vi "Array2DLastNColumns.vi"(2 "Array in":dbl[][](array[numeric]), 3 "N":i32=950) -> (1 "Array out":dbl[][](array[numeric]))   [LabVIEW 2014]
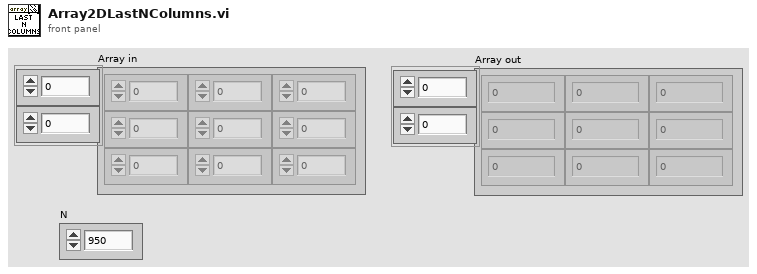
[diagram p1: front panel]
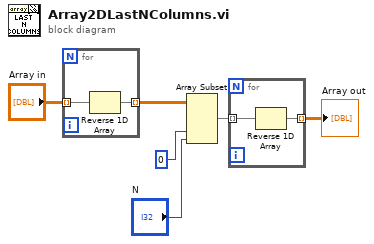
[diagram p0: block diagram]
diagram:
  n1 = for {
    tunnel: "Array in" -> [w8] mode=indexing
    tunnel: [w7] -> w4 mode=indexing
    n2 = Reverse 1D Array(array=w8) -> (reversed array=w7:dbl[])
  }
  n3 = Array Subset(array=w4, index (col)=0 ("index"), length (col)="N") -> (w5:dbl[][])  [unwired: 2 in]
  n4 = for {
    tunnel: w5 -> [w10] mode=indexing
    tunnel: [w9] -> w6 mode=indexing
    n5 = Reverse 1D Array(array=w10) -> (reversed array=w9:dbl[])
  }
  "Array out" <- w6
